vi "TestAdvanceTable.vi"() -> ()   [LabVIEW 2015, in "ActorManagement.lvlib"]
uses:
  ActorManagement.lvlib
  AdvanceTable/AdvanceTable.lvclass
  MakeTableItem/ConcreteTableItem.lvclass
  Scroll/Scroller.lvclass
panel:
  in  "stop":bool
  in  "data":T1
  in  "Items":T2
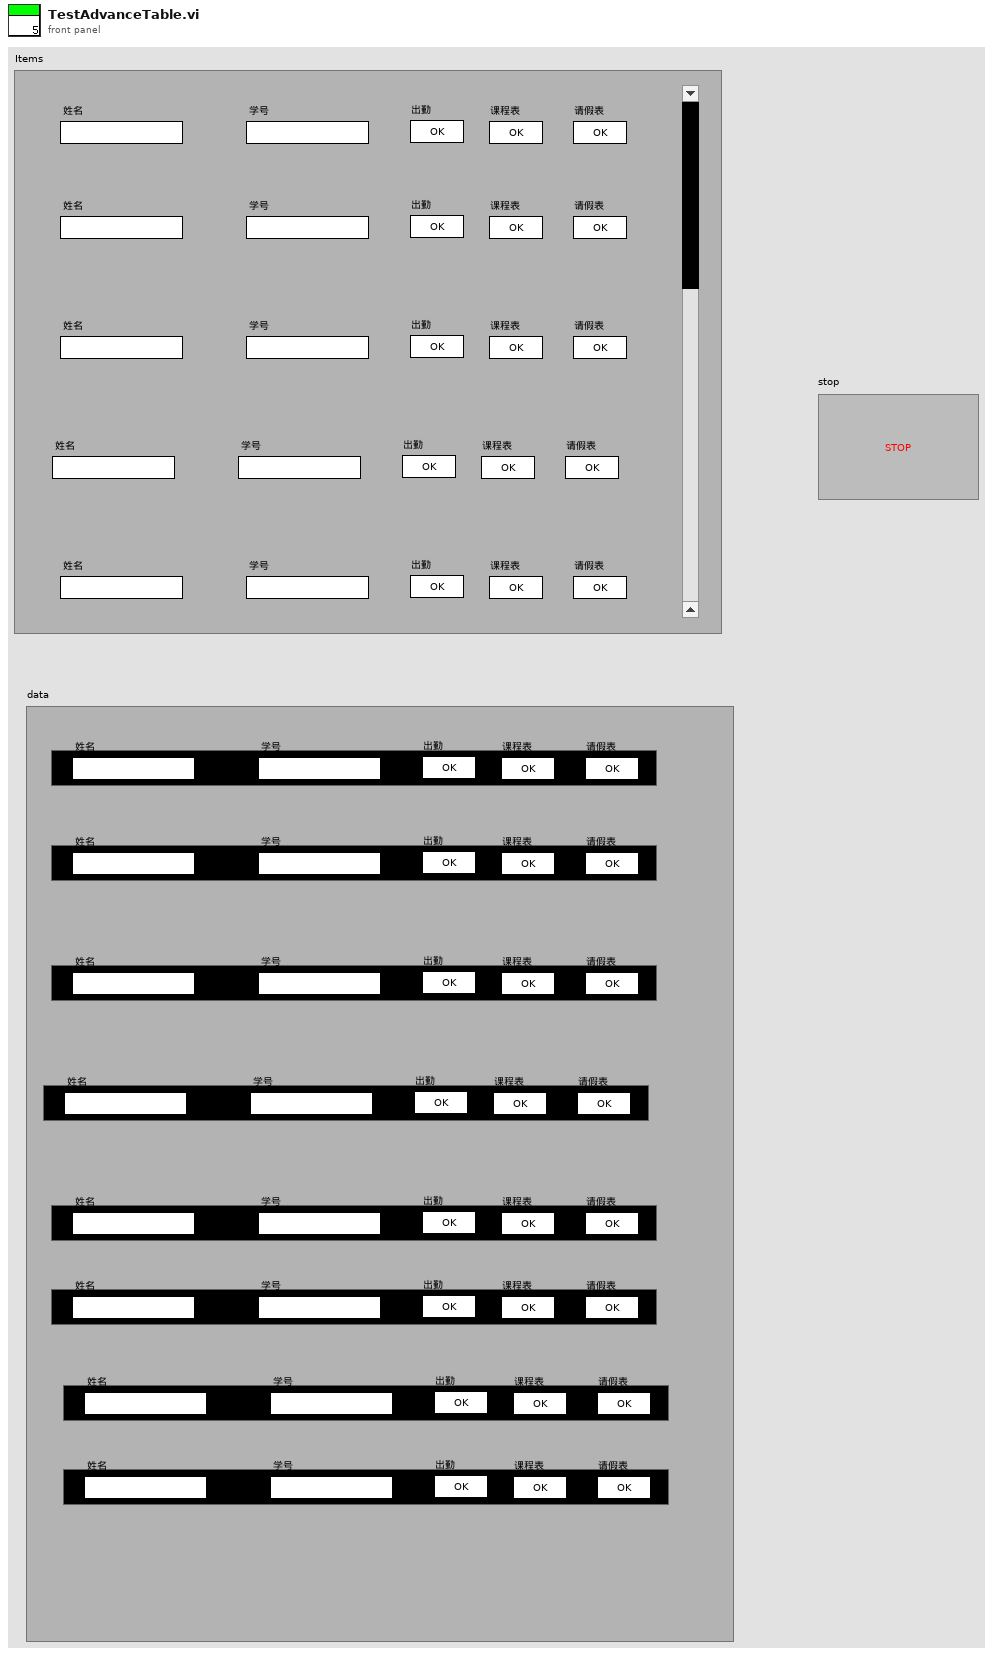
[diagram p1: front panel]
types:
  T1 = cluster{"Item":cluster{"背景色":u32, "姓名":string, "学号":string, "出勤":bool, "课程表":bool, "请假表":bool}, "Item 2":cluster{"背景色":u32, "姓名":string, "学号":string, "出勤":bool, "课程表":bool, "请假表":bool}, "Item 3":cluster{"背景色":u32, "姓名":string, "学号":string, "出勤":bool, "课程表":bool, "请假表":bool}, "Item 4":cluster{"背景色":u32, "姓名":string, "学号":string, "出勤":bool, "课程表":bool, "请假表":bool}, "Item 5":cluster{"背景色":u32, "姓名":string, "学号":string, "出勤":bool, "课程表":bool, "请假表":bool}, "Item 6":cluster{"背景色":u32, "姓名":string, "学号":string, "出勤":bool, "课程表":bool, "请假表":bool}, "Item 7":cluster{"背景色":u32, "姓名":string, "学号":string, "出勤":bool, "课程表":bool, "请假表":bool}, "Item 8":cluster{"背景色":u32, "姓名":string, "学号":string, "出勤":bool, "课程表":bool, "请假表":bool}}
  T2 = cluster{"Item 1":cluster{"背景色":u32, "姓名":string, "学号":string, "出勤":bool, "课程表":bool, "请假表":bool}, "Item 2":cluster{"背景色":u32, "姓名":string, "学号":string, "出勤":bool, "课程表":bool, "请假表":bool}, "Item 3":cluster{"背景色":u32, "姓名":string, "学号":string, "出勤":bool, "课程表":bool, "请假表":bool}, "Item 4":cluster{"背景色":u32, "姓名":string, "学号":string, "出勤":bool, "课程表":bool, "请假表":bool}, "Item 5":cluster{"背景色":u32, "姓名":string, "学号":string, "出勤":bool, "课程表":bool, "请假表":bool}, "Scrollbar":i32}
  T3 = cluster{"背景色":u32, "姓名":string, "学号":string, "出勤":bool, "课程表":bool, "请假表":bool}[]
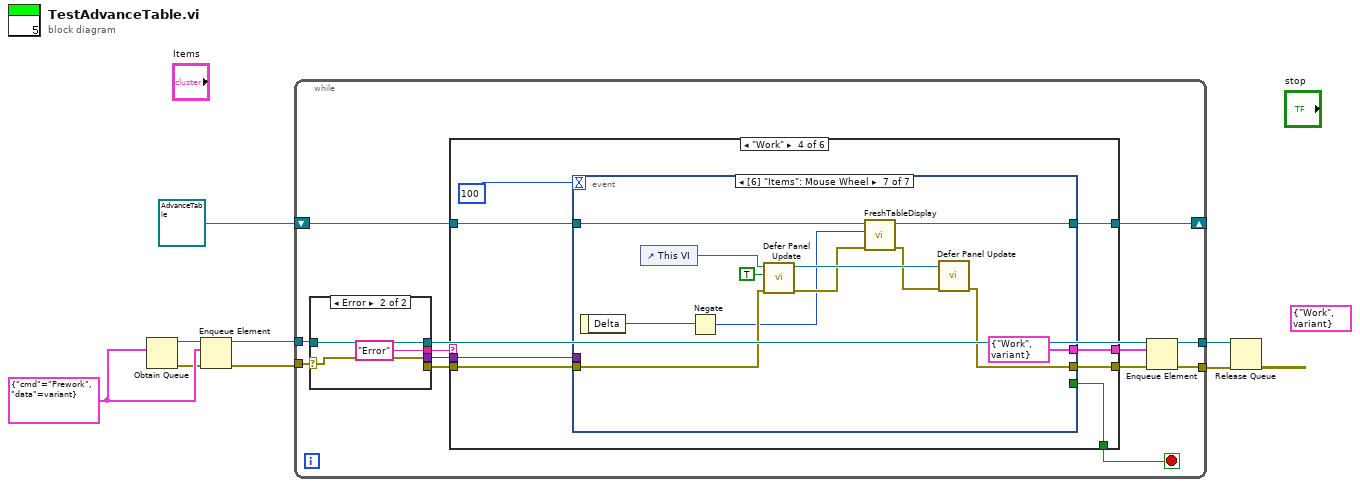
[diagram p0: block diagram]
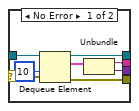
[diagram p2: hidden frame]
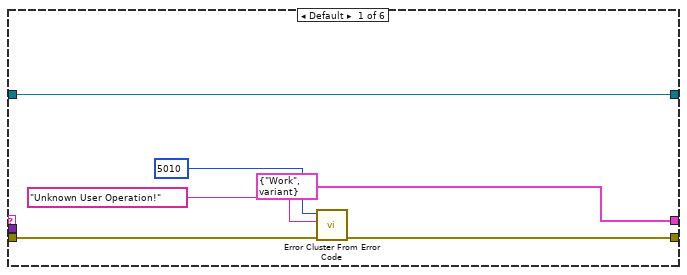
[diagram p3: hidden frame]
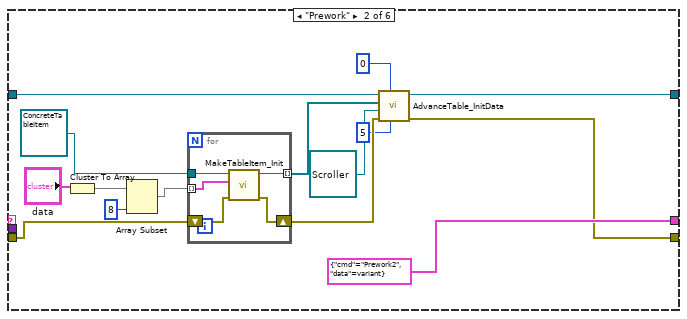
[diagram p4: hidden frame]
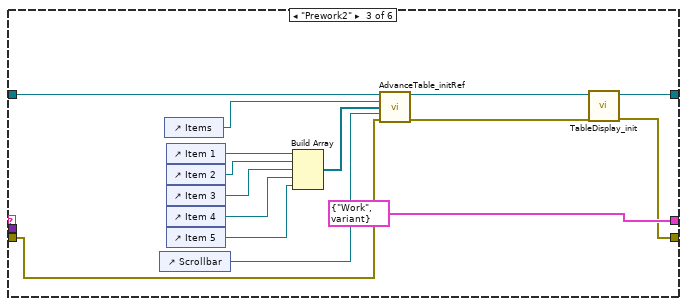
[diagram p5: hidden frame]
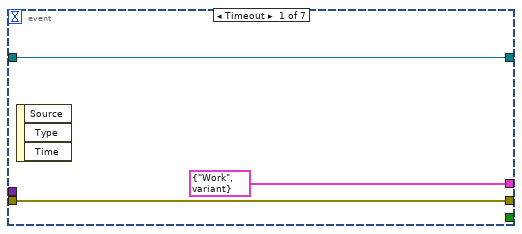
[diagram p6: hidden frame]
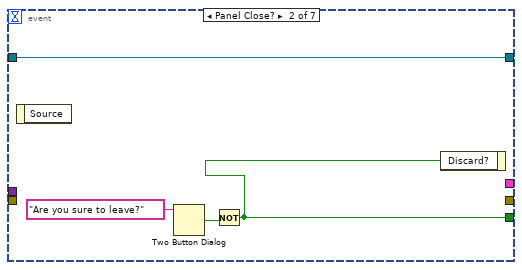
[diagram p7: hidden frame]
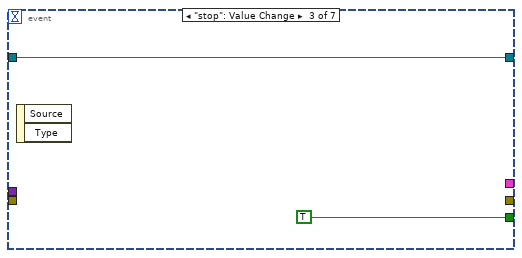
[diagram p8: hidden frame]
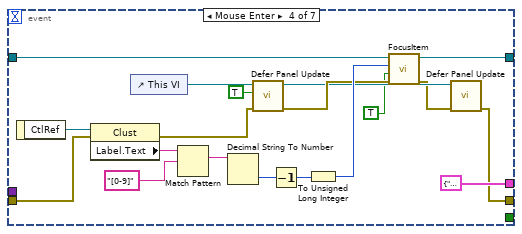
[diagram p9: hidden frame]
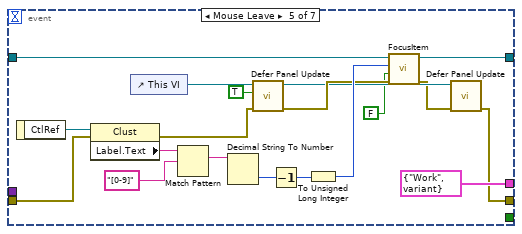
[diagram p10: hidden frame]
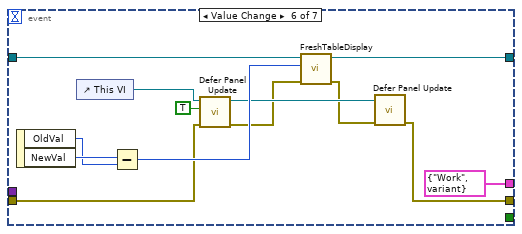
[diagram p11: hidden frame]
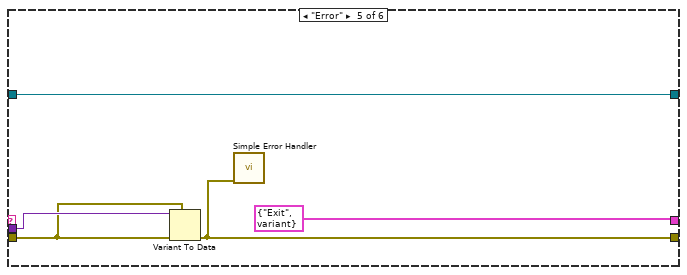
[diagram p12: hidden frame]
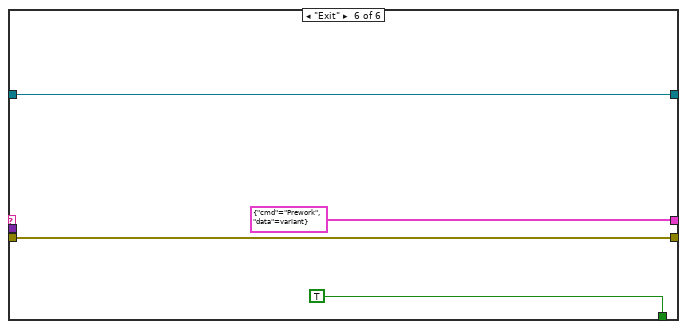
[diagram p13: hidden frame]
diagram:
  (unwired) cluster{"cmd":string, "data":variant} {"cmd"="Work", "data"=variant}
  w6 = cluster{"cmd":string, "data":variant} {"cmd"="Prework", "data"=variant}
  n1 = Obtain Queue(element data type=w6) -> (queue out=w2:refnum<queue>, error out=w3:errorcluster)  [unwired: 4 in, 1 out]
  n2 = Enqueue Element(queue=w2, element=w6, error in (no error)=w3) -> (queue out=w4:refnum<queue>, error out=w5:errorcluster)  [unwired: 1 in, 1 out]
  n3 = while {
    tunnel: w4 -> [w20]
    tunnel: w5 -> [w21]
    tunnel: [w12] -> w7
    tunnel: [w11] -> w8
    shift-right: [w9] -> _
    shift-left: refnum<class "AdvanceTable.lvclass"> refnum ("ActorManagement.lvlib:AdvanceTable") -> [w10]
    stop <- w13 stop-if-true
    n4 = case shown="Error" w21 {
      selector: w21 -> [w28 w31]
      tunnel: w20 -> [w29 w32]
      tunnel: [w26 w32] -> w18
      tunnel: [w25 _] -> w16
      tunnel: [w23 "Error" ("cmd")] -> w17
      tunnel: [w22 w31] -> w19
      frame No Error {
        n5 = Dequeue Element(queue=w29, timeout in ms (-1)=10, error in (no error)=w28) -> (queue out=w26:refnum<queue>, element=w24:cluster{"cmd":string, "data":variant}, error out=w25:errorcluster)  [unwired: 1 out]
        n6 = Unbundle(w24) -> ("cmd"=w23:string, "data"=w22:variant)
      }
      frame Error {
      }
    }
    n7 = case shown="\"Work\"" w17 {
      tunnel: w19 -> [_ _ _ w81 w158 _]
      tunnel: w16 -> [w35 w49 w64 w80 w157 w162]
      tunnel: [cluster{"cmd":string, "data":variant} {"cmd"="Work", "data"=variant} cluster{"cmd":string, "data":variant} {"cmd"="Prework2", "data"=variant} cluster{"cmd":string, "data":variant} {"cmd"="Work", "data"=variant} w78 cluster{"cmd":string, "data":variant} {"cmd"="Exit", "data"=variant} cluster{"cmd":string, "data":variant} {"cmd"="Prework", "data"=variant}] -> w15
      tunnel: [w36 w43 w60 w77 w155 w162] -> w14
      tunnel: [_ _ _ w76 _ TRUE] -> w13
      tunnel: w10 -> [w33 w52 w68 w75 w154 w159]
      tunnel: [w33 w42 w59 w74 w154 w159] -> w9
      frame Default {
        n8 = call <vilib>:"Error Cluster From Error Code.vi"("error in (no error)"=w35, "error message (\"\")"="Unknown User Operation!" ("error message (\"\")"), "error code (0)"=5010) -> ("error out"=w36:errorcluster)  [unwired: 6 in]
      }
      frame "Prework" {
        n9 = Cluster To Array(cluster="data") -> (array=w41:T3)
        n10 = Array Subset(array=w41, length=8) -> (w39:T3)  [unwired: 1 in]
        n11 = for {
          tunnel: w39 -> [w57] mode=indexing
          tunnel: refnum<class "ConcreteTableItem.lvclass"> refnum ("object in") -> [w58]
          shift-right: [w55] -> w45
          shift-left: w49 -> [w56]
          tunnel: [w54] -> w48 mode=indexing
          n12 = call "MakeTableItem_Init.vi"("error in (no error)"=w56, "Item"=w57, "object in"=w58) -> ("error out"=w55:errorcluster, "object out"=w54:refnum<class "ConcreteTableItem.lvclass">)  [unwired: 7 in]
        }
        n13 = call "AdvanceTable_InitData.vi"("NumInPage"=u32 5 ("NumOfDisplay"), "NumOfUnsaw"=u32 0, "error in (no error)"=w45, "Scroller.lvclass"=refnum<class "Scroller.lvclass"> refnum, "Items"=w48, "object in"=w52) -> ("error out"=w43:errorcluster, "object out"=w42:refnum<class "AdvanceTable.lvclass">)  [unwired: 4 in]
      }
      frame "Prework2" {
        n14 = control-ref of="Scrollbar"() -> (w65:refnum<vi>)
        n15 = control-ref of="Items"() -> (w67:refnum<vi>)
        n16 = control-ref of="Item 1"() -> (w73:refnum<vi>)
        n17 = control-ref of="Item 2"() -> (w72:refnum<vi>)
        n18 = control-ref of="Item 3"() -> (w71:refnum<vi>)
        n19 = control-ref of="Item 4"() -> (w70:refnum<vi>)
        n20 = control-ref of="Item 5"() -> (w69:refnum<vi>)
        n21 = Build Array(w73, w72, w71, w70, w69) -> (w66:refnum<vi>[])
        n22 = call "AdvanceTable_initRef.vi"("AdvanceTable in"=w68, "AdvanceTable"=w67, "ItemsArray"=w66, "RefOfScroll"=w65, "error in (no error)"=w64) -> ("AdvanceTable out"=w62:refnum<class "AdvanceTable.lvclass">, "error out"=w61:errorcluster)  [unwired: 9 in]
        n23 = call "TableDisplay_init.vi"("error in (no error)"=w61, "AdvanceTable in"=w62) -> ("error out"=w60:errorcluster, "AdvanceTable out"=w59:refnum<class "AdvanceTable.lvclass">)  [unwired: 8 in]
      }
      frame "Work" {
        n24 = event shown="[6] \"Items\": Mouse Wheel" {
          selector: _ -> [_ _ _ _ _ _ _]
          dyn-events: _ -> [_ _ _ _ _ _ _]
          timeout: 100 -> [_ _ _ _ _ _ _]
          tunnel: w81 -> [_ _ _ _ _ _ _]
          tunnel: w80 -> [w83 _ _ w107 w126 w132 w147]
          tunnel: [cluster{"cmd":string, "data":variant} {"cmd"="Work", "data"=variant} _ _ cluster{"cmd":string, "data":variant} {"cmd"="Work", "data"=variant} cluster{"cmd":string, "data":variant} {"cmd"="Work", "data"=variant} cluster{"cmd":string, "data":variant} {"cmd"="Work", "data"=variant} cluster{"cmd":string, "data":variant} {"cmd"="Work", "data"=variant}] -> w78
          tunnel: [w83 _ _ w92 w111 w131 w146] -> w77
          tunnel: [_ w86 TRUE _ _ _ _] -> w76
          tunnel: w75 -> [w82 w85 w89 w109 w128 w138 w153]
          tunnel: [w82 w85 w89 w102 w121 w129 w144] -> w74
          event Timeout {
            n25 = event-data() -> ()  [unwired: 1 in, 3 out]
          }
          event Panel Close? {
            n26 = event-data() -> ()  [unwired: 1 in, 1 out]
            n27 = Two Button Dialog(message="Are you sure to leave?") -> (T button?=w87:bool)  [unwired: 2 in]
            n28 = Not(x=w87) -> (.not. x?=w86:bool)
            n29 = event-data("Discard?"=w86) -> ()  [unwired: 1 in, 1 out]
          }
          event "stop": Value Change {
            n30 = event-data() -> ()  [unwired: 1 in, 2 out]
          }
          event "Items.Item 1", "Items.Item 2", "Items.Item 3", "Items.Item 4", "Items.Item 5": Mouse Enter {
            n31 = event-data() -> ("CtlRef"=w108:refnum<vi>)  [unwired: 1 in]
            n32 = property class="Clust"(reference=w108, error in=w107) -> (error out=w95:errorcluster, "Label.Text"=w106:string)  [unwired: 1 out]
            n33 = control-ref of="This VI"() -> (w98:refnum<vi>)
            n34 = Match Pattern(string=w106, regular expression="[0-9]") -> (match substring=w104:string)  [unwired: 1 in, 3 out]
            n35 = Decimal String To Number(string=w104) -> (number=w103:i32)  [unwired: 2 in, 1 out]
            n36 = call "Defer Panel Update.vi"("error in (no error)"=w95, "Defer Panel Updates(false)"=TRUE, "VI in"=w98) -> ("error out"=w96:errorcluster, "VI  out"=w94:refnum<vi>)  [unwired: 7 in]
            n37 = Decrement(x=w103) -> (x-1=w100:i32)
            n38 = To Unsigned Long Integer(number=w100) -> (unsigned 32bit integer=w99:u32)
            n39 = call "FocusItem.vi"("error in (no error)"=w96, "Focus?(False)"=TRUE, "Index"=w99, "AdvanceTable in"=w109) -> ("error out"=w93:errorcluster, "AdvanceTable out"=w102:refnum<class "AdvanceTable.lvclass">)  [unwired: 6 in]
            n40 = call "Defer Panel Update.vi"("error in (no error)"=w93, "VI in"=w94) -> ("error out"=w92:errorcluster)  [unwired: 8 in, 1 out]
          }
          event "Items.Item 1", "Items.Item 2", "Items.Item 3", "Items.Item 4", "Items.Item 5": Mouse Leave {
            n41 = event-data() -> ("CtlRef"=w127:refnum<vi>)  [unwired: 1 in]
            n42 = property class="Clust"(reference=w127, error in=w126) -> (error out=w114:errorcluster, "Label.Text"=w125:string)  [unwired: 1 out]
            n43 = control-ref of="This VI"() -> (w117:refnum<vi>)
            n44 = Match Pattern(string=w125, regular expression="[0-9]") -> (match substring=w123:string)  [unwired: 1 in, 3 out]
            n45 = Decimal String To Number(string=w123) -> (number=w122:i32)  [unwired: 2 in, 1 out]
            n46 = call "Defer Panel Update.vi"("error in (no error)"=w114, "Defer Panel Updates(false)"=TRUE, "VI in"=w117) -> ("error out"=w115:errorcluster, "VI  out"=w113:refnum<vi>)  [unwired: 7 in]
            n47 = Decrement(x=w122) -> (x-1=w119:i32)
            n48 = To Unsigned Long Integer(number=w119) -> (unsigned 32bit integer=w118:u32)
            n49 = call "FocusItem.vi"("error in (no error)"=w115, "Focus?(False)"=FALSE, "Index"=w118, "AdvanceTable in"=w128) -> ("error out"=w112:errorcluster, "AdvanceTable out"=w121:refnum<class "AdvanceTable.lvclass">)  [unwired: 6 in]
            n50 = call "Defer Panel Update.vi"("error in (no error)"=w112, "VI in"=w113) -> ("error out"=w111:errorcluster)  [unwired: 8 in, 1 out]
          }
          event Value Change {
            n51 = event-data() -> ("OldVal"=w140:i32, "NewVal"=w141:i32)  [unwired: 1 in]
            n52 = control-ref of="This VI"() -> (w133:refnum<vi>)
            n53 = Subtract(x=w141, y=w140) -> (x-y=w139:i32)
            n54 = call "Defer Panel Update.vi"("error in (no error)"=w132, "Defer Panel Updates(false)"=TRUE, "VI in"=w133) -> ("error out"=w136:errorcluster, "VI  out"=w137:refnum<vi>)  [unwired: 7 in]
            n55 = call "FreshTableDisplay.vi"("error in (no error)"=w136, "IndexDelta"=w139, "AdvanceTable in"=w138) -> ("error out"=w135:errorcluster, "AdvanceTable out"=w129:refnum<class "AdvanceTable.lvclass">)  [unwired: 7 in]
            n56 = call "Defer Panel Update.vi"("error in (no error)"=w135, "VI in"=w137) -> ("error out"=w131:errorcluster)  [unwired: 8 in, 1 out]
          }
          event "Items": Mouse Wheel {
            n57 = event-data() -> ("Delta"=w143:i32)  [unwired: 1 in]
            n58 = control-ref of="This VI"() -> (w148:refnum<vi>)
            n59 = Negate(x=w143) -> (-x=w142:i32)
            n60 = call "Defer Panel Update.vi"("error in (no error)"=w147, "Defer Panel Updates(false)"=TRUE, "VI in"=w148) -> ("error out"=w151:errorcluster, "VI  out"=w152:refnum<vi>)  [unwired: 7 in]
            n61 = call "FreshTableDisplay.vi"("error in (no error)"=w151, "IndexDelta"=w142, "AdvanceTable in"=w153) -> ("error out"=w150:errorcluster, "AdvanceTable out"=w144:refnum<class "AdvanceTable.lvclass">)  [unwired: 7 in]
            n62 = call "Defer Panel Update.vi"("error in (no error)"=w150, "VI in"=w152) -> ("error out"=w146:errorcluster)  [unwired: 8 in, 1 out]
          }
        }
      }
      frame "Error" {
        n63 = Variant To Data(error in=w157, type=w157, Variant=w158) -> (error out=w155:errorcluster)  [unwired: 1 out]
        n64 = call <vilib>:"Simple Error Handler.vi"("error in (no error)"=w155) -> ()  [unwired: 4 in, 5 out]
      }
      frame "Exit" {
      }
    }
    n65 = Enqueue Element(queue=w18, element=w15, error in (no error)=w14) -> (queue out=w12:refnum<queue>, error out=w11:errorcluster)  [unwired: 1 in, 1 out]
  }
  n66 = Release Queue(queue=w7, error in (no error)=w8) -> ()  [unwired: 1 in, 3 out]
